vi "7.vi"() -> ()   [LabVIEW 2017]
uses:
  <vilib>/Utility/file.llb/Read Delimited Spreadsheet (DBL).vi
  <vilib>/Analysis/NI_AALBase.lvlib
panel:
  out "波形图表":dbl[][](graph)
  in  "cycles":dbl=1.0 caption="周期" format="%0.2f"
  out "all rows":dbl[][](array[numeric]) caption="所有行"
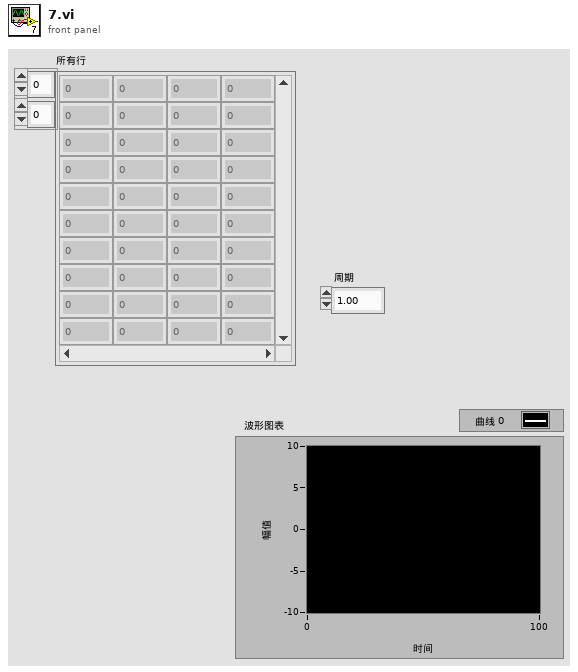
[diagram p1: front panel]
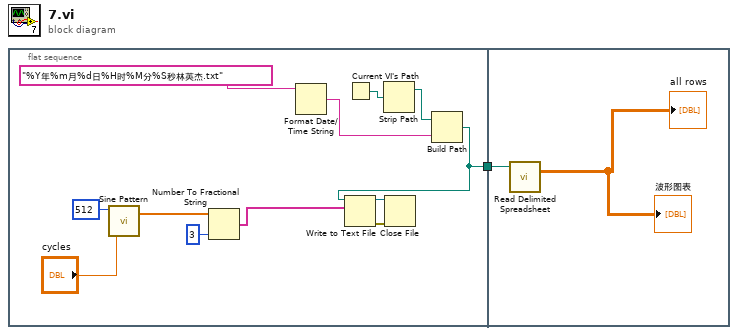
[diagram p0: block diagram]
diagram:
  n1 = flat-sequence {
    tunnel: [w5] -> w1
    tunnel: w1 -> [w15]
    frame #0 {
      n2 = call <vilib>:"Sine Pattern.vi"("cycles"="cycles", "samples"=512) -> ("Sinusoidal Pattern"=w8:dbl[])  [unwired: 2 in, 1 out]
      n3 = Number To Fractional String(number=w8, precision (6)=i16 3 ("精度(6)")) -> (F-format string=w6:string[])  [unwired: 2 in]
      n4 = Format Date/Time String(time format string (%c)="%Y年%m月%d日%H时%M分%S秒林英杰.txt" ("时间格式字符串(%c)")) -> (date/time string=w10:string)  [unwired: 2 in]
      n5 = Current VI's Path() -> (path=w12:path)
      n6 = Strip Path(path=w12) -> (stripped path=w11:path)  [unwired: 1 out]
      n7 = Build Path(base path=w11, name or relative path=w10) -> (appended path=w5:path)
      n8 = Write to Text File(file (use dialog)=w5, text=w6) -> (refnum out=w3:refnum<file>, error out=w4:errorcluster)  [unwired: 2 in, 1 out]
      n9 = Close File(refnum=w3, error in=w4) -> ()  [unwired: 2 out]
    }
    frame #1 {
      n10 = call-poly <vilib>:"Read Delimited Spreadsheet.vi"("file path (dialog if empty)"=w15) -> ("all rows"=→"all rows" →"波形图表":dbl[][])  [unwired: 9 in, 5 out]
    }
  }
